vi "DSF.Engine.Framework.Active Transfer Groups.vi"(8 "error in (no error)":errorcluster, 10 "Plugin index in":i32, 11 "Framework in":refnum<class "Framework.lvclass">) -> (0 "error out":errorcluster, 1 "active Transfer Group indicies":i32[](array[numeric]), 2 "Plugin index out":i32, 3 "Framework out":refnum<class "Framework.lvclass">)   [LabVIEW 2016, in "DSF.Engine.lvlib" / "Framework.lvclass"]
uses:
  Framework.lvclass
  Framework.lvclass/Framework.ctl
  Plugin/Plugin.lvclass/Plugin.ctl
  Transfer/DSF.Engine.Transfer Group.lvclass/DSF.Engine.Transfer Group.ctl
  DSF.Engine.Framework.Get Plugins.vi
  Transfer/DSF.Engine.Transfer Group.lvclass
  Shared/Classes/Timing/DSF.Shared.Timing.lvclass
  Plugin/Plugin.lvclass
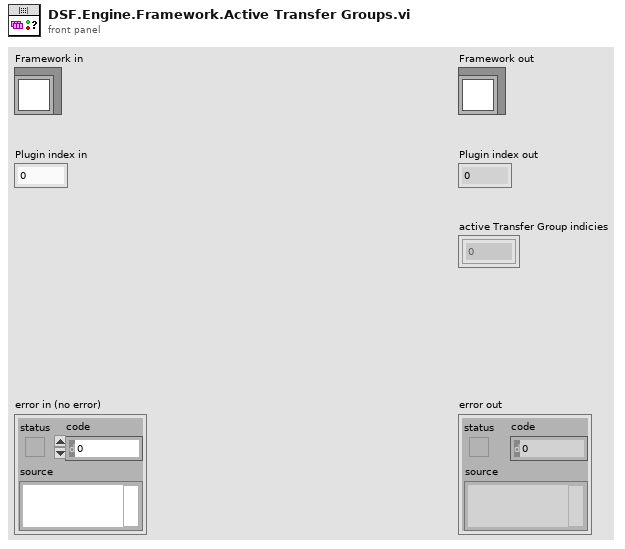
[diagram p1: front panel]
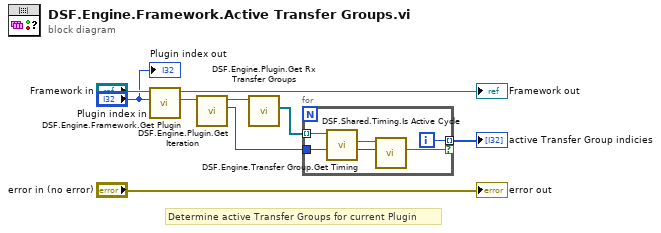
[diagram p0: block diagram]
diagram:
  # "Determine active Transfer Groups for current Plugin"
  n1 = call "DSF.Engine.Framework.Get Plugin.vi"("index"="Plugin index in", "Framework in"="Framework in") -> ("Plugin"=w6:refnum<class "Plugin.lvclass">, "Framework out"=→"Framework out":refnum<class "Framework.lvclass">)  [unwired: 8 in]
  n2 = call "DSF.Engine.Plugin.Get Iteration.vi"("Plugin in"=w6) -> ("iteration"=w8:u64, "Plugin out"=w7:refnum<class "Plugin.lvclass">)  [unwired: 9 in]
  n3 = call "DSF.Engine.Plugin.Get Rx Transfer Groups.vi"("Plugin in"=w7) -> ("Rx Transfer Groups"=w5:refnum<class "DSF.Engine.Transfer Group.lvclass">[])  [unwired: 9 in, 1 out]
  n4 = for {
    tunnel: w5 -> [w14] mode=indexing
    tunnel: w8 -> [w12]
    tunnel: [w11] -> w9 mode=indexing if=w10
    i -> [w11]
    n5 = call "DSF.Engine.Transfer Group.Get Timing.vi"("Transfer Group in"=w14) -> ("Timing"=w13:refnum<class "DSF.Shared.Timing.lvclass">)  [unwired: 9 in, 1 out]
    n6 = call "DSF.Shared.Timing.Is Active Cycle.vi"("iteration"=w12, "Timing in"=w13) -> ("active?"=w10:bool)  [unwired: 8 in, 1 out]
  }
  "active Transfer Group indicies" <- w9
  "error out" <- "error in (no error)"
  "Plugin index out" <- "Plugin index in"
